vi "Write Cell.vi"(8 "error in (no error)":errorcluster, 10 "Cell":u8, 11 "Change Laser Frequency CMD in":refnum<class "Change Laser Frequency CMD.lvclass">) -> (0 "error out":errorcluster, 3 "Change Laser Frequency CMD out":refnum<class "Change Laser Frequency CMD.lvclass">)   [LabVIEW 2016, in "gPAS Library.lvlib" / "Change Laser Frequency CMD.lvclass"]
uses:
  Change Laser Frequency CMD.lvclass
  Change Laser Frequency CMD.lvclass/Change Laser Frequency CMD.ctl
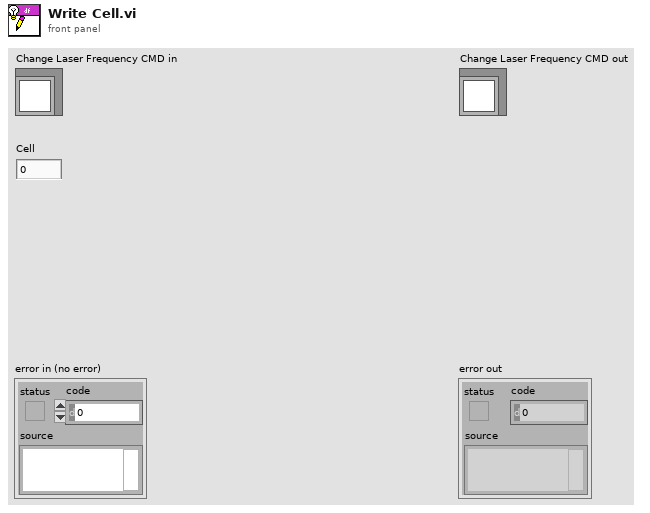
[diagram p1: front panel]
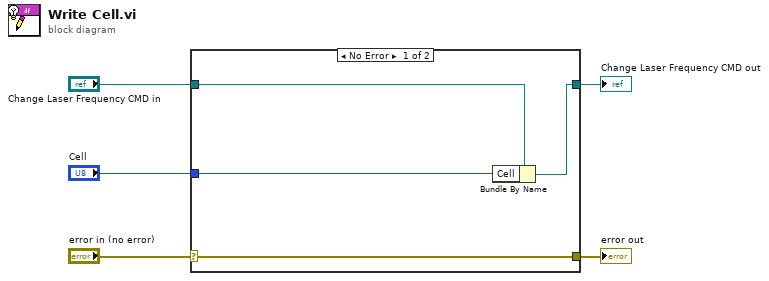
[diagram p0: block diagram]
diagram:
  n1 = case shown="No Error" "error in (no error)" {
    selector: "error in (no error)" -> [w9 w10]
    tunnel: [w9 w10] -> w4
    tunnel: [w7 w11] -> w2
    tunnel: "Change Laser Frequency CMD in" -> [w8 w11]
    tunnel: "Cell" -> [w6 _]
    frame No Error {
      n2 = Bundle By Name(cluster=w8, "Cell"=w6) -> (w7:refnum<class "Change Laser Frequency CMD.lvclass">)
    }
    frame Error {
    }
  }
  "error out" <- w4
  "Change Laser Frequency CMD out" <- w2
